vi "straight.vi"() -> ()   [LabVIEW 2009]
uses:
  <vilib>/Analysis/NI_AALBase.lvlib
panel:
  out "歪み率(%)":dbl
  in  "ホワイトノイズの最大振幅":dbl
  out "DC":cluster{dbl[], dbl[]}(graph)
  out "AC":cluster{dbl[], dbl[]}(graph)
  in  "カットオフ周波数(Hz)":dbl
  in  "Q":dbl
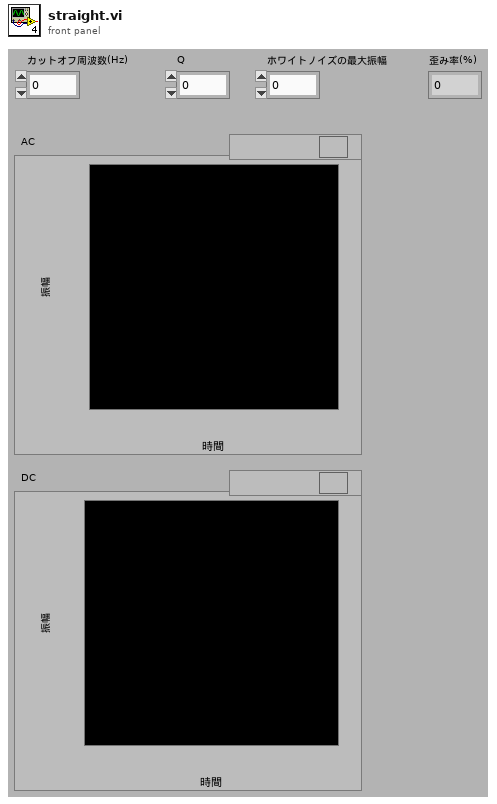
[diagram p1: front panel]
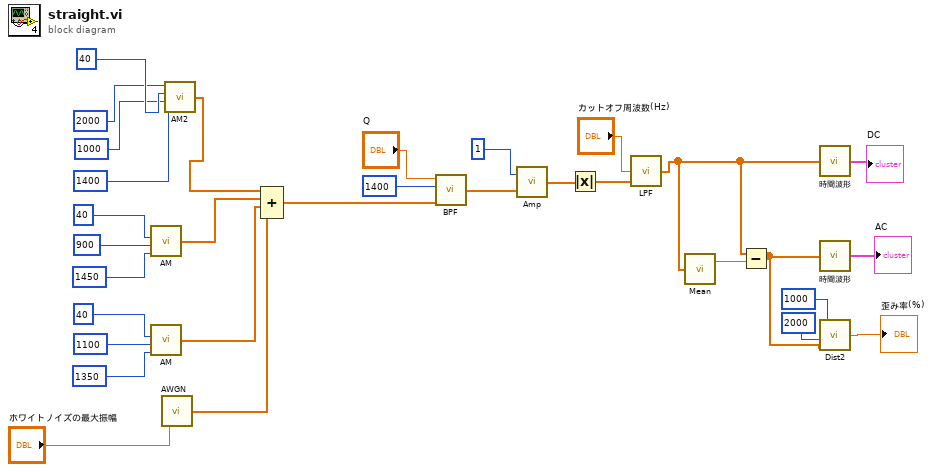
[diagram p0: block diagram]
diagram:
  n1 = call "AM.vi"("変調度 [%]"=40, "変調周波数 [Hz]"=900, "搬送波周波数 [kHz]"=1450) -> ("変調波"=w25:dbl[])  [unwired: 2 in]
  n2 = call "AM.vi"("変調度 [%]"=40, "変調周波数 [Hz]"=1100, "搬送波周波数 [kHz]"=1350) -> ("変調波"=w24:dbl[])  [unwired: 2 in]
  n3 = call "AWGN.vi"("振幅値"="ホワイトノイズの最大振幅") -> ("出力"=w23:dbl[])
  n4 = call "AM2.vi"("搬送波周波数 [kHz]"=1400, "変調周波数1 [Hz]"=1000, "変調度 [%]"=40, "変調周波数2 [Hz]"=2000) -> ("変調波"=w1:dbl[])  [unwired: 2 in]
  n5 = Compound Arithmetic op=ADD(w1, w25, w24, w23) -> (w22:dbl[])
  n6 = call "BPF.vi"("X"=w22, "中心周波数 [kHz]"=1400, "Q"="Q") -> ("BPF出力"=w20:dbl[])  [unwired: 1 in]
  n7 = call "Amp.vi"("入力"=w20, "増幅率"=1) -> ("出力"=w17:dbl[])
  n8 = Absolute Value(x=w17) -> (abs(x)=w16:dbl[])
  n9 = call "LPF.vi"("入力"=w16, "カットオフ周波数 [Hz]"="カットオフ周波数(Hz)") -> ("LPF出力"=w13:dbl[])  [unwired: 1 in]
  n10 = call <vilib>:"Mean.vi"("X"=w13) -> ("mean"=w14:dbl)  [unwired: 1 out]
  n11 = Subtract(x=w13, y=w14) -> (x-y=w9:dbl[])
  n12 = call "時間波形.vi"("入力"=w13) -> ("時間波形"=→"DC":cluster{dbl[], dbl[]})
  n13 = call "時間波形.vi"("入力"=w9) -> ("時間波形"=→"AC":cluster{dbl[], dbl[]})
  n14 = call "Dist2.vi"("入力"=w9, "基本周波数1 [Hz]"=2000, "基本周波数2 [Hz]"=1000) -> ("ひずみ率"=→"歪み率(%)":dbl)  [unwired: 1 in]
